vi "DMSS.main.vi"() -> ()   [LabVIEW 2014, in "DMSServer.lvlib"]
doc: "descriptionHelpStart\nThe DomainManagementServer publishes information about a CS controls domain.\n\nIt publishes four types of DIM services\n1) \"DOMAINNAME_Tasks@NODENAME\": A list of taks. Each task has a name, command line parameters and options. There is one service for each task.\n\n2) \"DOMAINNAME_CSSystems\": A list of CS systems inside the domain.\n\n3) \"DOMAINNAME_Nodes\": A list of all nodes of the domain\n\n4) \"DOMAINNAME_Info\": A service for entertaining users.\n\nFor more information please refer to\nhttp://wiki.gsi.de/cgi-bin/view/CSframework/DomainManagementSystem\ndescriptionHelpStop\n\nHistory: 16-FEB-2006, Dietrich Beck\n\nCopyright (C)\nGesellschaft für Schwerionenforschung, GSI\nPlanckstr. 1\n64291 Darmstadt\nGermany\n\nContact: D.Beck@gsi.de \n\nThis program is free software; you can redistribute it and/or modify it under the terms of the \nGNU General Public License as published by the Free Software Foundation; either version 2 of the license, or (at your option) any later version.\n\nThis program is distributed in the hope that it will be useful, but WITHOUT ANY WARRANTY; without even the implied warranty of MERCHANTABILITY or FITNESS FOR A PARTICULAR PURPOSE. See the GNU General License for more details (http://www.gnu.org).\n\nGesellschaft für Schwerionenforschung, GSI\nPlanckstr. 1, 64291 Darmstadt, Germany\nFor all questions and ideas contact D. Beck.\nLast update: 16-DEC-2005\n\n\nmenuHelpStart\nFile\n==\n- \"Load Settings\" loads a setting (*.xml) file, containing the information about a domain.\n\n- \"Save Settings\" saves the actual configuration to a setting (*.xml) file.\n\n- \"Quit (don't kill proce)\" exits this program without killing the processes marked \"kill on exit\"\n\n- \"Exit (kill procs)\" exits this program and kills the processes marked \"kill on exit\".\n\nHelp\n===\n- \"Show Description\" shows the description about this program.\n\n- \"Explain Menus\" shows this explanation\n\n- \"About LabVIEW\" shows information about LabVIEW.\n\nmenuHelpStop"
uses:
  DMSServer.lvlib
  DMSS.process_type.ctl
  DomainManagementUtils/DMSU.restart_mode.ctl
  CSlibraries/UtilityLib/UtilityLib.valueStatus.ctl
  DMSS.node_type.ctl
  CSlibraries/UtilityLib/UtilityLib.helpType.ctl
  <vilib>/Utility/xml.llb/Read From XML File(array).vi
  <vilib>/Utility/xml.llb/Write to XML File(string).vi
  CSlibraries-extern/DimLVEvent/LVDimInterface/LVDimInterface.lvlib
  DomainManagementUtils/DMSUtils.lvlib
  CSlibraries/UtilityLib/UtilityLib.lvlib
panel:
  in  "nodes":cluster{"nodeName":string, "processes":T1[]}[](array[cluster]) {"processes"."restartMode" items=["UNKNOWN", "MANUAL", "ONCE", "ALWAYS", "KILL", "SHUTDOWN"]}
  in  "updateDomain":bool
  in  "sendMessage":bool
  in  "domainMessage":string="hello world :-)\n"
  in  "Messages":i32(listbox)=-1
  in  "setDomain":bool
  in  "selectNode":u16(ring)
  in  "DomainName":string="KSTest"
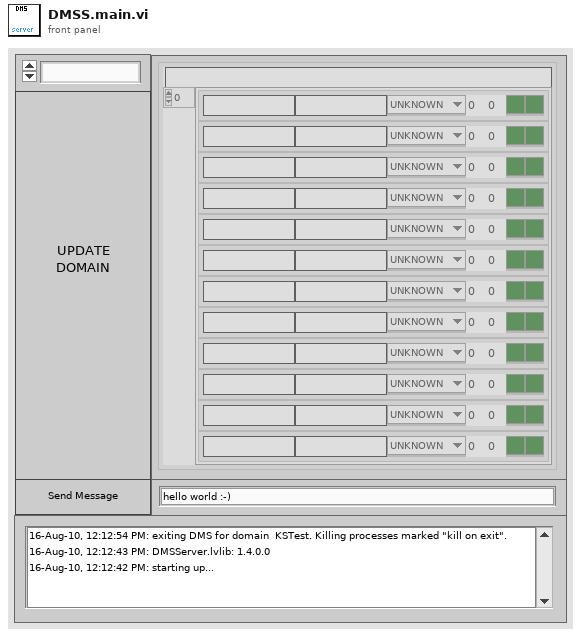
[diagram p1: front panel]
types:
  T1 = typedef "DMSServer.lvlib/DMSS.process_type.ctl" = cluster{"imageName":string, "argumentString":string, "restartMode":T2, "nOfRestart":i32, "resetRestartTimer":i32, "killOnExit":bool, "csSystem":bool}
  T2 = typedef "DMSUtils.lvlib/DMSU.restart_mode.ctl" = u16
  T3 = typedef "UtilityLib.lvlib/UtilityLib.valueStatus.ctl" = enum16{"no info available", "stand by/off", "on", "warning", "alarm/malfunction", "not implemented", "user action required", "important information", "system default", "control default", "indicator default", "button default"}
  T4 = typedef "DMSServer.lvlib/DMSS.node_type.ctl" = cluster{"nodeName":string, "processes":T1[]}
  T5 = enum16{"AddMessage", "AddErrorMessage", "GetMessages"}
  T6 = typedef "UtilityLib.lvlib/UtilityLib.helpType.ctl" = enum16{"unknown", "menu", "description", "about", "special0", "special1", "special2"}
  T7 = enum32{"invalid app kind", "Development System", "Run Time System", "Student Edition", "Embedded LabVIEW", "Evaluation", "Custom"}
  T8 = cluster{"elementBackground":u32, "elementBackground":u32}
  T9 = cluster{"elementBackground":u32, "elementBackground":u32}[]
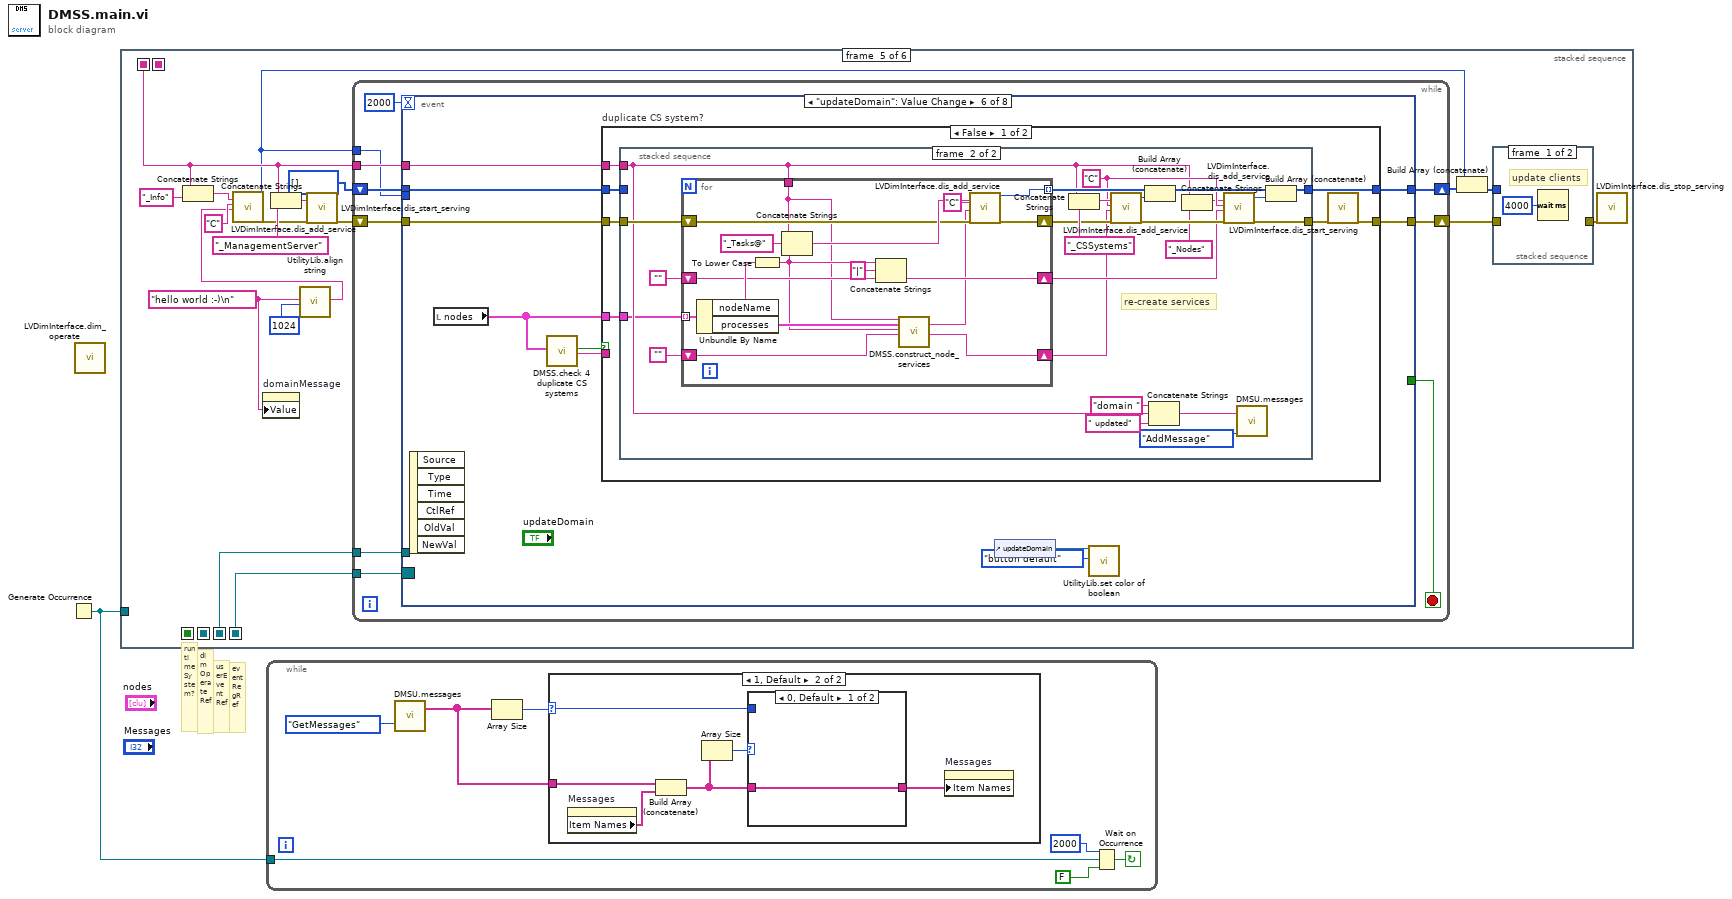
[diagram p0: block diagram]
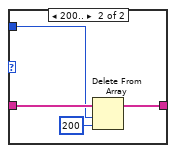
[diagram p3: hidden frame]
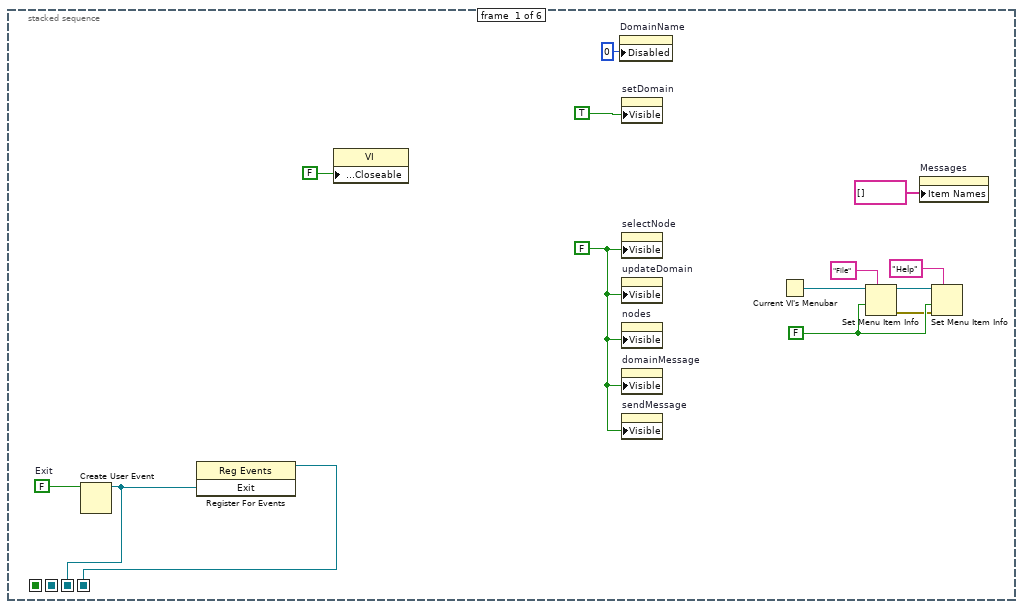
[diagram p4: hidden frame]
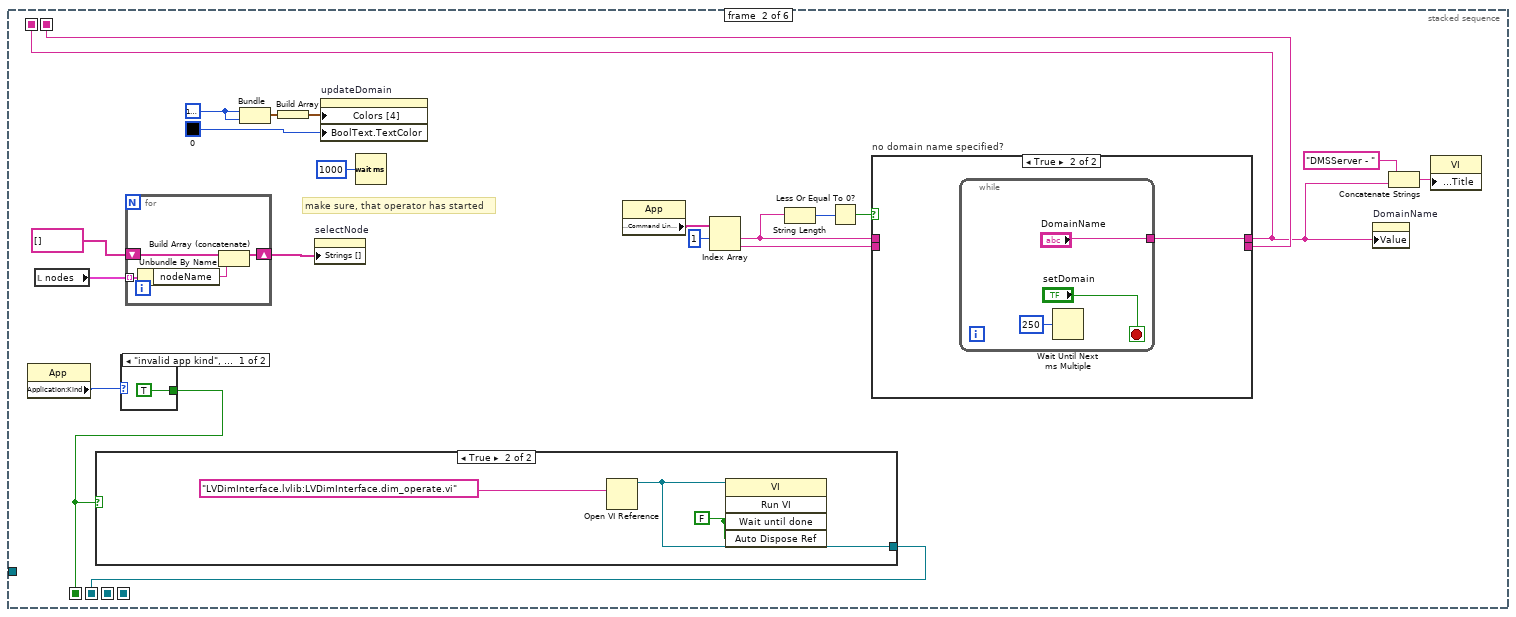
[diagram p5: hidden frame]
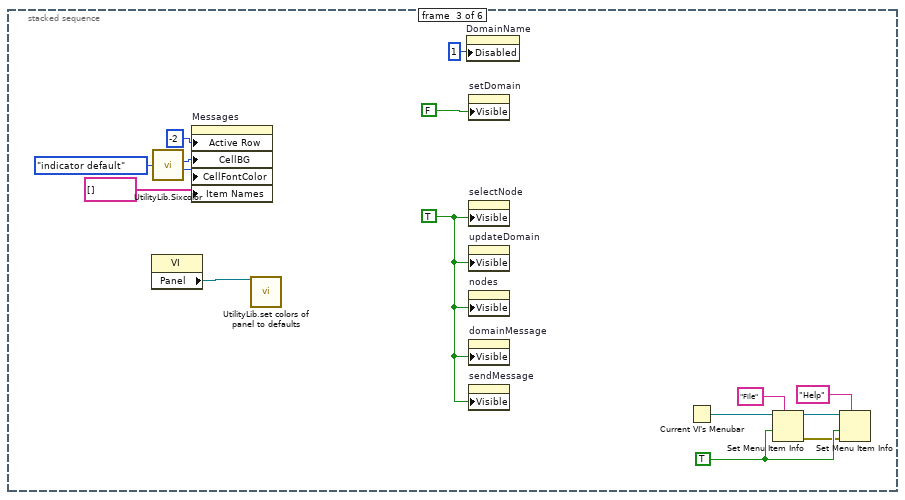
[diagram p9: hidden frame]
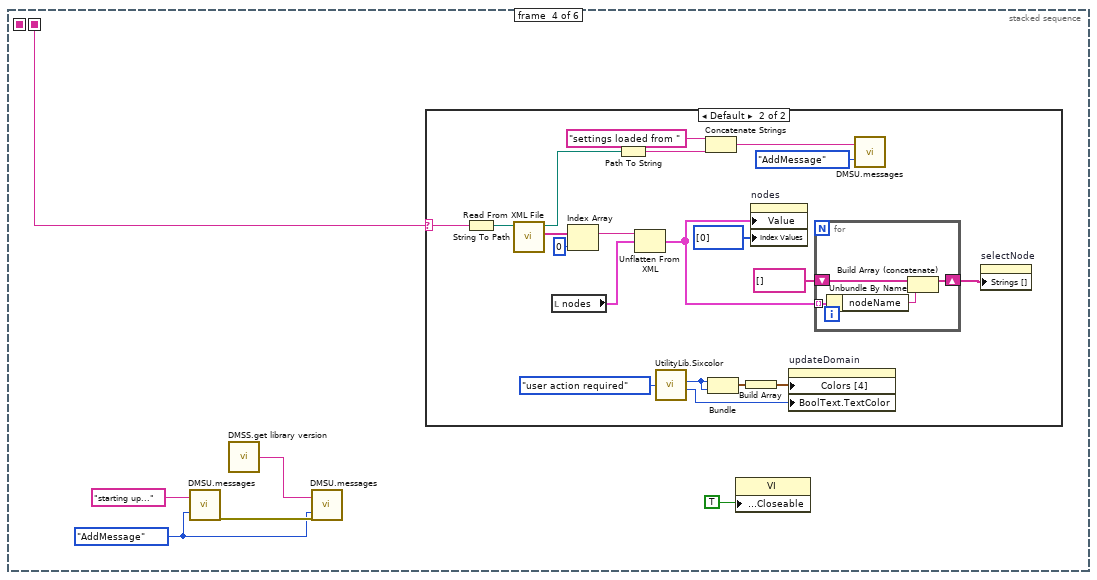
[diagram p10: hidden frame]
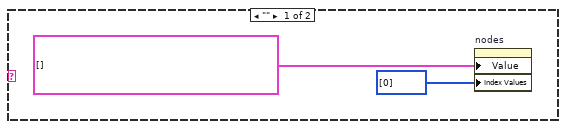
[diagram p11: hidden frame]
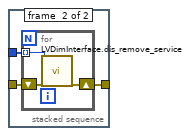
[diagram p12: hidden frame]
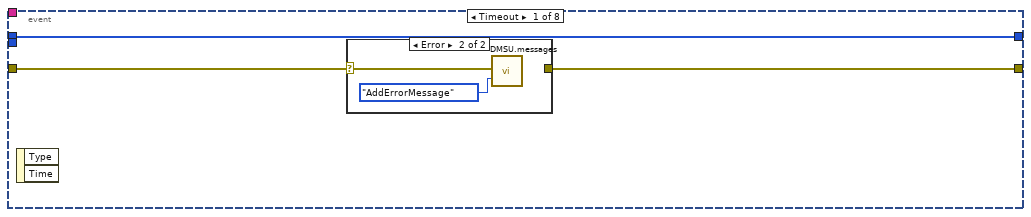
[diagram p13: hidden frame]
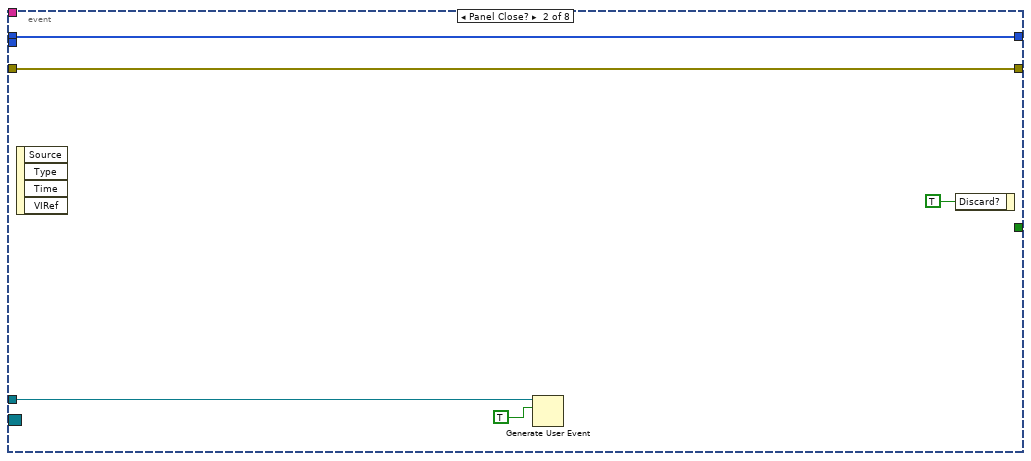
[diagram p15: hidden frame]
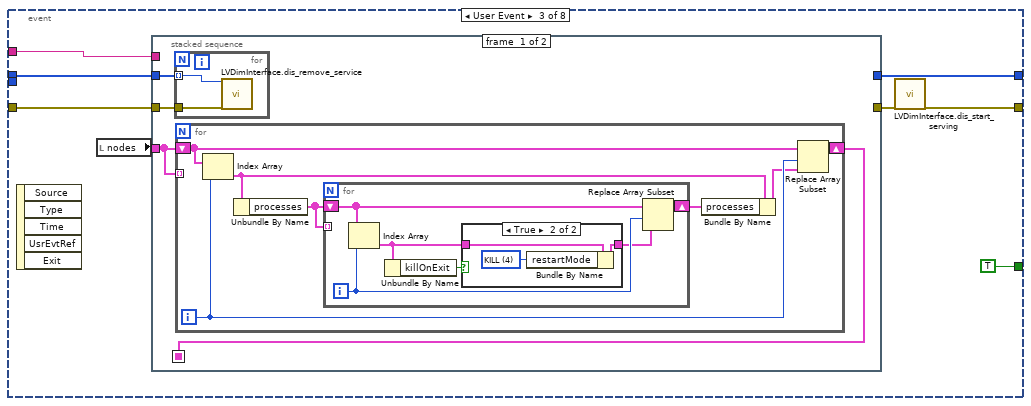
[diagram p16: hidden frame]
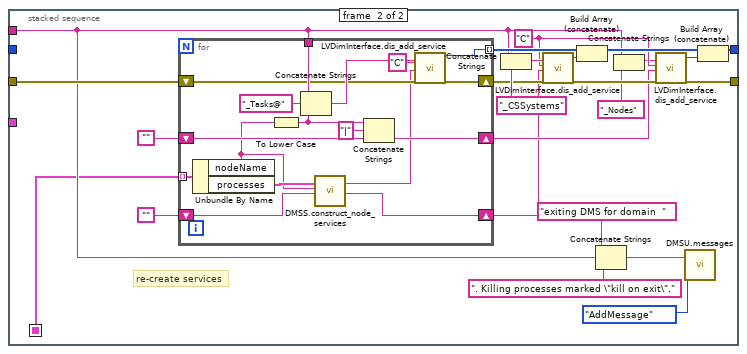
[diagram p18: hidden frame]
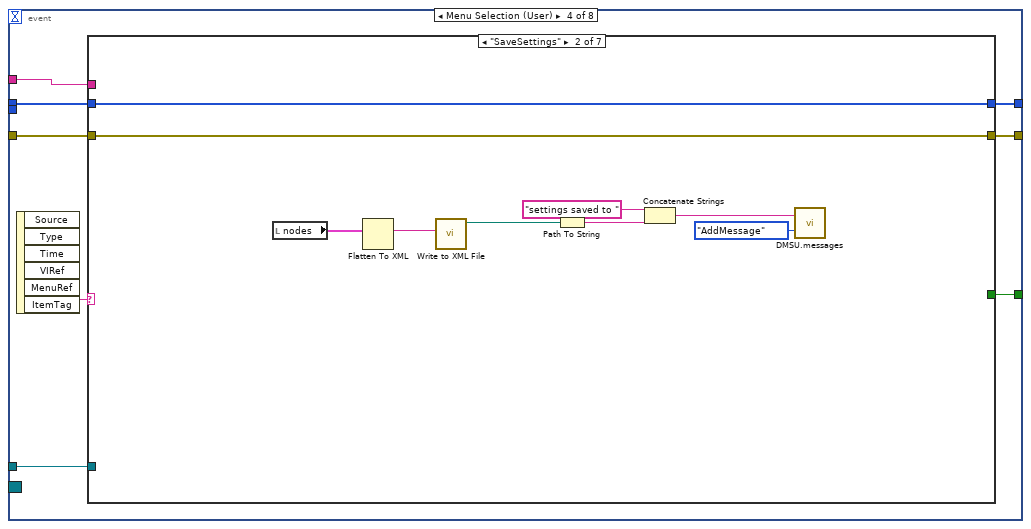
[diagram p19: hidden frame]
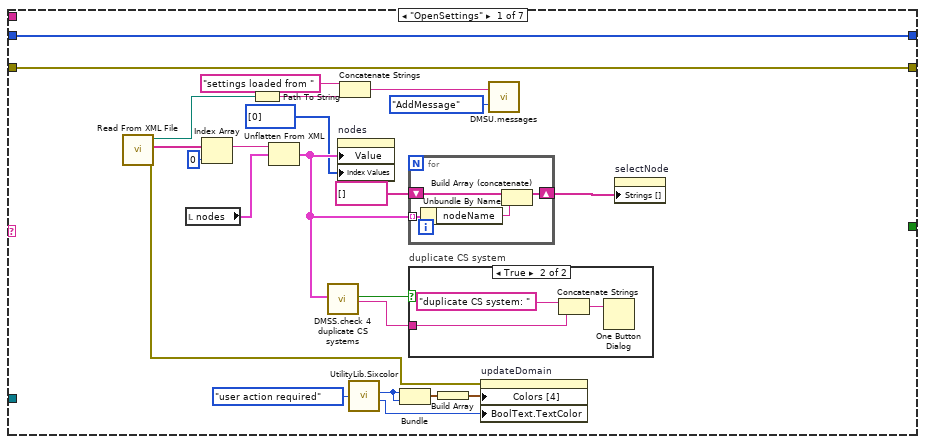
[diagram p20: hidden frame]
diagram:
  # "eventRegRef"
  # "userEventRef"
  # "dimOperateRef"
  # "runtimeSystem?"
  n1 = Generate Occurrence() -> (w1:refnum<k4>)
  n2 = call "LVDimInterface.dim_operate.vi"() -> ()  [unwired: 20 in]
  n3 = stacked-sequence {
    seq-local: [_ w20 _ _ _ _] -> [_ _ _ _ w108 _]
    seq-local: [_ w27 _ _ _ _] -> [_ _ _ _ _ w410]
    seq-local: [_ w25 _ _ _ _] -> [_ _ _ _ _ w411]
    seq-local: [_ w23 _ _ _ _] -> [_ _ _ w71 _ _]
    seq-local: [w6 _ _ _ _ _] -> [_ _ _ _ w102 _]
    seq-local: [w5 _ _ _ _ _] -> [_ _ _ _ w103 _]
    tunnel: w1 -> [_ _ _ _ _ w412]
    frame #0 {
      w7 = FALSE  # Exit
      w13 = FALSE ("enabled")
      w2 = FALSE
      n4 = Create User Event(user event datatype=w7) -> (user event=w6:refnum<user-event>)  [unwired: 1 in, 1 out]
      n5 = register-events(w6) -> (reference out=w5:refnum<event-registration>)  [unwired: 2 in, 1 out]
      n6 = property class="VI"("Front Panel.Closeable"=FALSE ("Front Panel Window:Closeable")) -> ()  [unwired: 2 in, 2 out]
      n7 = property on="DomainName" class="Str"("Disabled"=u8 0) -> ()  [unwired: 2 in, 2 out]
      n8 = property on="setDomain" class="Bool"("Visible"=TRUE) -> ()  [unwired: 2 in, 2 out]
      n9 = property on="selectNode" class="Ring (strict)"("Visible"=w2) -> ()  [unwired: 2 in, 2 out]
      n10 = property on="updateDomain" class="Bool"("Visible"=w2) -> ()  [unwired: 2 in, 2 out]
      n11 = property on="nodes" class="Arr (strict)"("Visible"=w2) -> ()  [unwired: 2 in, 2 out]
      n12 = property on="domainMessage" class="Str"("Visible"=w2) -> ()  [unwired: 2 in, 2 out]
      n13 = property on="sendMessage" class="Bool"("Visible"=w2) -> ()  [unwired: 2 in, 2 out]
      n14 = Current VI's Menubar() -> (w12:refnum<k9>)
      n15 = Set Menu Item Info(7:"File" ("item name"), 9:w13, 11:w12) -> (0:w11:errorcluster, 3:w10:refnum<k9>)  [unwired: 4 in]
      n16 = property on="Messages" class="LstBox (strict)"("Item Names"=string[] []) -> ()  [unwired: 2 in, 2 out]
      n17 = Set Menu Item Info(7:"Help" ("item name"), 8:w11, 9:w13, 11:w10) -> ()  [unwired: 3 in, 2 out]
    }
    frame #1 {
      w17 = u32 16777238 ("Color Box")
      # "make sure, that operator has started"
      n18 = property on="Property Node" class="App"() -> ("Application:Kind"=w26:T7)  [unwired: 2 in, 2 out]
      n19 = local read "nodes"() -> (w34:cluster{"nodeName":string, "processes":T1[]}[])
      n20 = case shown="\"invalid app kind\", Default" w26 {
        tunnel: [TRUE _] -> w25
        frame "invalid app kind", Default {
        }
        frame "Development System" {
        }
      }
      n21 = case shown="True" w25 {
        tunnel: [_ w39] -> w27
        frame False {
        }
        frame True {
          w40 = FALSE ("Wait until done")
          n22 = Open VI Reference(vi path="LVDimInterface.lvlib:LVDimInterface.dim_operate.vi") -> (vi reference=w39:refnum<vi>)  [unwired: 5 in, 1 out]
          n23 = invoke on="Invoke Node" class="VI" method="Run VI"(reference=w39, "Wait until done"=w40, "Auto Dispose Ref"=w40) -> ()  [unwired: 2 in, 5 out]
        }
      }
      n24 = for {
        shift-right: [w49] -> w33
        shift-left: string[] [] -> [w48]
        tunnel: w34 -> [w50] mode=indexing
        n25 = Unbundle By Name(w50) -> ("nodeName"=w47:string)
        n26 = Build Array (concatenate)(w48, w47) -> (w49:string[])
      }
      n27 = Bundle("Color Box"=w17, "Color Box"=w17) -> (w19:cluster{"Color Box":u32, "Color Box":u32})  [unwired: 1 in]
      n28 = Build Array(w19) -> (w18:cluster{"Color Box":u32, "Color Box":u32}[])
      n29 = property on="selectNode" class="Ring (strict)"("Strings []"=w33) -> ()  [unwired: 2 in, 2 out]
      n30 = property on="updateDomain" class="Bool"("Colors [4]"=w18, "BoolText.TextColor"=u32 0 ("Color Box")) -> ()  [unwired: 2 in, 2 out]
      n31 = Wait (ms)(milliseconds to wait=u32 1000) -> ()  [unwired: 1 out]
      n32 = property on="Property Node" class="App"() -> ("Application:Command Line Arguments"=w32:string[])  [unwired: 2 in, 2 out]
      n33 = Index Array(array=w32, index #1=1 ("index")) -> (element #1=w28:string, element #2=w24:string)  [unwired: 1 in]
      n34 = String Length(string=w28) -> (length=w30:i32)
      n35 = Less Or Equal To 0?(x=w30) -> (x <= 0?=w29:bool)
      n36 = case "no domain name specified?" shown="True" w29 {
        tunnel: [w42 w43] -> w20
        tunnel: w28 -> [w42 _]
        tunnel: [w41 _] -> w23
        tunnel: w24 -> [w41 _]
        frame False {
        }
        frame True {
          n37 = while {
            tunnel: ["DomainName"] -> w43
            stop <- "setDomain" stop-if-true
            n38 = Wait Until Next ms Multiple(millisecond multiple=u32 250) -> ()  [unwired: 1 out]
          }
        }
      }
      n39 = property on="DomainName" class="Str"("Value"=w20) -> ()  [unwired: 2 in, 2 out]
      n40 = Concatenate Strings("DMSServer - " ("string"), w20) -> (w22:string)
      n41 = property on="Property Node" class="VI"("Front Panel.Title"=w22) -> ()  [unwired: 2 in, 2 out]
    }
    frame #2 {
      w64 = TRUE ("enabled")
      w51 = TRUE
      n42 = property on="Property Node" class="VI"() -> ("Panel"=w53:refnum<vi>)  [unwired: 2 in, 2 out]
      n43 = call "UtilityLib.Sixcolor.vi"("State"=UtilityLib.valueStatus."indicator default") -> ("elementBackground"=w57:u32, "elementText"=w56:u32)  [unwired: 2 in, 2 out]
      n44 = property on="Messages" class="LstBox (strict)"("Active Row"=-2 ("Active Row:Active Row Number"), "CellBG"=w57, "CellFontColor"=w56, "Item Names"=string[] []) -> ()  [unwired: 2 in, 2 out]
      n45 = call "UtilityLib.set colors of panel to defaults.vi"("Front Panel"=w53) -> ()  [unwired: 18 in, 1 out]
      n46 = property on="DomainName" class="Str"("Disabled"=u8 1) -> ()  [unwired: 2 in, 2 out]
      n47 = property on="setDomain" class="Bool"("Visible"=FALSE) -> ()  [unwired: 2 in, 2 out]
      n48 = property on="selectNode" class="Ring (strict)"("Visible"=w51) -> ()  [unwired: 2 in, 2 out]
      n49 = property on="updateDomain" class="Bool"("Visible"=w51) -> ()  [unwired: 2 in, 2 out]
      n50 = property on="nodes" class="Arr (strict)"("Visible"=w51) -> ()  [unwired: 2 in, 2 out]
      n51 = property on="domainMessage" class="Str"("Visible"=w51) -> ()  [unwired: 2 in, 2 out]
      n52 = property on="sendMessage" class="Bool"("Visible"=w51) -> ()  [unwired: 2 in, 2 out]
      n53 = Current VI's Menubar() -> (w63:refnum<k9>)
      n54 = Set Menu Item Info(7:"File" ("item name"), 9:w64, 11:w63) -> (0:w62:errorcluster, 3:w61:refnum<k9>)  [unwired: 4 in]
      n55 = Set Menu Item Info(7:"Help" ("item name"), 8:w62, 9:w64, 11:w61) -> ()  [unwired: 3 in, 2 out]
    }
    frame #3 {
      w66 = T5."AddMessage" ("Action")
      n56 = call "DMSU.messages.vi"("message"="starting up...", "Action"=w66) -> ("error out"=w68:errorcluster)  [unwired: 16 in, 1 out]
      n57 = call "DMSS.get library version.vi"() -> ("nameAndVersion"=w67:string)  [unwired: 1 in]
      n58 = call "DMSU.messages.vi"("message"=w67, "Action"=w66, "error in (no error)"=w68) -> ()  [unwired: 15 in, 2 out]
      n59 = case shown="Default" w71 {
        selector: w71 -> [_ w81]
        frame "" {
          n60 = property on="nodes" class="Arr (strict)"("Value"=T4[] [] ("nodes"), "Index Values"=u32[] [0]) -> ()  [unwired: 2 in, 2 out]
        }
        frame Default {
          n61 = String To Path(string=w81) -> (path=w82:path)
          n62 = call-poly <vilib>:"Read From XML File.vi"("XML File Path"=w82) -> ("XML Elements"=w93:string[], "XML File Path(duplicate)"=w83:path)  [unwired: 8 in, 1 out]
          n63 = local read "nodes"() -> (w88:cluster{"nodeName":string, "processes":T1[]}[])
          n64 = Index Array(array=w93, index=0) -> (element=w91:string)
          n65 = Path To String(path=w83) -> (string=w85:string)
          n66 = Unflatten From XML(xml string=w91, type=w88) -> (value=w74:cluster{"nodeName":string, "processes":T1[]}[])  [unwired: 1 in, 1 out]
          n67 = call "UtilityLib.Sixcolor.vi"("State"=UtilityLib.valueStatus."user action required") -> ("elementBackground"=w77:u32, "elementText"=w76:u32)  [unwired: 2 in, 2 out]
          n68 = Concatenate Strings("settings loaded from " ("message"), w85) -> (w84:string)
          n69 = Bundle("elementBackground"=w77, "elementBackground"=w77) -> (w79:T8)  [unwired: 1 in]
          n70 = Build Array(w79) -> (w78:T9)
          n71 = property on="nodes" class="Arr (strict)"("Value"=w74, "Index Values"=u32[] [0]) -> ()  [unwired: 2 in, 2 out]
          n72 = property on="updateDomain" class="Bool"("Colors [4]"=w78, "BoolText.TextColor"=w76) -> ()  [unwired: 2 in, 2 out]
          n73 = for {
            shift-right: [w96] -> w89
            shift-left: string[] [] -> [w95]
            tunnel: w74 -> [w97] mode=indexing
            n74 = Unbundle By Name(w97) -> ("nodeName"=w94:string)
            n75 = Build Array (concatenate)(w95, w94) -> (w96:string[])
          }
          n76 = call "DMSU.messages.vi"("message"=w84, "Action"=T5."AddMessage") -> ()  [unwired: 16 in, 2 out]
          n77 = property on="selectNode" class="Ring (strict)"("Strings []"=w89) -> ()  [unwired: 2 in, 2 out]
        }
      }
      n78 = property class="VI"("Front Panel.Closeable"=TRUE ("Front Panel Window:Closeable")) -> ()  [unwired: 2 in, 2 out]
    }
    frame #4 {
      w98 = "hello world :-)\n" ("data")
      n79 = Concatenate Strings(w108, "_Info" ("string")) -> (w110:string)
      n80 = property on="domainMessage" class="Str"("Value"=w98) -> ()  [unwired: 2 in, 2 out]
      n81 = Concatenate Strings(w108, "_ManagementServer" ("string")) -> (w116:string)
      n82 = call "UtilityLib.align string.vi"("stringIn"=w98, "stringLength (80)"=u16 1024) -> ("stringOut"=w100:string)  [unwired: 16 in, 1 out]
      n83 = call "LVDimInterface.dis_add_service.vi"("serviceName"=w110, "typeDescriptor"="C", "data"=w100) -> ("my_serviceID"=w101:i32, "error out"=w107:errorcluster)  [unwired: 15 in]
      n84 = call "LVDimInterface.dis_start_serving.vi"("serverName"=w116, "error in (no error)"=w107) -> ("error out"=w114:errorcluster)  [unwired: 16 in, 1 out]
      n85 = while {
        tunnel: w108 -> [w130]
        shift-right: [w129] -> w105
        shift-left: i32[] [] -> [w128]
        shift-right: [w131] -> w113
        shift-left: w114 -> [w132]
        tunnel: w103 -> [w126]
        tunnel: w102 -> [w125]
        tunnel: w101 -> [w124]
        stop <- w133 stop-if-true
        n86 = event shown="[5] \"updateDomain\": Value Change" {
          selector: w126 -> [_ _ _ _ _ _ _ _]
          dyn-events: _ -> [_ _ _ _ _ _ _ _]
          timeout: 2000 -> [_ _ _ _ _ _ _ _]
          tunnel: [_ _ TRUE w219 _ _ _ _] -> w133
          tunnel: w132 -> [w135 w142 w147 w220 w288 w305 w367 w382]
          tunnel: [w134 w142 w145 w221 w288 w304 w367 w375] -> w131
          tunnel: w130 -> [_ _ w149 w218 _ w308 _ _]
          tunnel: [w136 w143 w146 w222 w291 w307 w368 w373] -> w129
          tunnel: w128 -> [w136 w143 w148 w223 w291 w306 w368 w374]
          tunnel: w125 -> [_ w140 _ w217 _ _ _ _]
          tunnel: w124 -> [_ _ _ _ _ _ _ w383]
          event Timeout {
            n87 = event-data() -> ()  [unwired: 1 in, 2 out]
            n88 = case shown="Error" w135 {
              selector: w135 -> [w137 w139]
              tunnel: [w137 _] -> w134
              frame No Error {
              }
              frame Error {
                n89 = call "DMSU.messages.vi"("errorMessage"=w139, "Action"=T5."AddErrorMessage") -> ()  [unwired: 16 in, 2 out]
              }
            }
          }
          event Panel Close? {
            n90 = event-data() -> ()  [unwired: 1 in, 4 out]
            n91 = Generate User Event(user event=w140, event data cluster=TRUE ("event data")) -> ()  [unwired: 2 in, 2 out]
            n92 = event-data ("Event Filter Node")("Discard?"=TRUE) -> ()  [unwired: 1 in, 1 out]
          }
          event User Event {
            n93 = event-data() -> ()  [unwired: 1 in, 5 out]
            n94 = local read "nodes"() -> (w150:cluster{"nodeName":string, "processes":T1[]}[])
            n95 = stacked-sequence {
              seq-local: [w153 _] -> [_ w176]
              tunnel: w149 -> [_ w177]
              tunnel: [_ w187] -> w146
              tunnel: w148 -> [w156 _]
              tunnel: [_ w190] -> w151
              tunnel: w147 -> [w155 w198]
              tunnel: w150 -> [w154 _]
              frame #0 {
                n96 = for {
                  tunnel: w156 -> [w175] mode=indexing
                  tunnel: w155 -> [w174]
                  n97 = call "LVDimInterface.dis_remove_service.vi"("my_serviceID"=w175, "error in (no error)"=w174) -> ()  [unwired: 17 in, 1 out]
                }
                n98 = for {
                  tunnel: w154 -> [_] mode=indexing
                  shift-right: [w161] -> w153
                  shift-left: w154 -> [w162]
                  i -> [w160]
                  n99 = Index Array(array=w162, index=w160) -> (element=w159:cluster{"nodeName":string, "processes":T1[]})
                  n100 = Unbundle By Name(w159) -> ("processes"=w163:T1[])
                  n101 = for {
                    tunnel: w163 -> [_] mode=indexing
                    shift-right: [w164] -> w158
                    shift-left: w163 -> [w168]
                    i -> [w167]
                    n102 = Index Array(array=w168, index=w167) -> (element=w166:T1)
                    n103 = Unbundle By Name(w166) -> ("killOnExit"=w169:bool)
                    n104 = case shown="True" w169 {
                      tunnel: [w170 w172] -> w165
                      tunnel: w166 -> [w170 w173]
                      frame False {
                      }
                      frame True {
                        w171 = T2 4 items=["UNKNOWN", "MANUAL", "ONCE", "ALWAYS", "KILL"] ("restartMode")
                        n105 = Bundle By Name(cluster=w173, "restartMode"=w171) -> (w172:T1)
                      }
                    }
                    n106 = Replace Array Subset(array=w168, new element=w165, index=w167) -> (w164:T1[])
                  }
                  n107 = Bundle By Name(cluster=w159, "processes"=w158) -> (w157:cluster{"nodeName":string, "processes":T1[]})
                  n108 = Replace Array Subset(array=w162, new element=w157, index=w160) -> (w161:cluster{"nodeName":string, "processes":T1[]}[])
                }
              }
              frame #1 {
                w184 = "C" ("typeDescriptor")
                # "re-create services"
                n109 = for {
                  tunnel: w176 -> [w216] mode=indexing
                  tunnel: w177 -> [w215]
                  tunnel: [w211] -> w194 mode=indexing
                  shift-right: [w201] -> w182
                  shift-left: "" ("Empty String Constant") -> [w202]
                  shift-right: [w210] -> w195
                  shift-left: w198 -> [w209]
                  shift-right: [w205] -> w185
                  shift-left: "" ("Empty String Constant") -> [w206]
                  n110 = Unbundle By Name(w216) -> ("nodeName"=w200:string, "processes"=w204:T1[])
                  n111 = To Lower Case(string=w200) -> (all lower case string=w207:string)
                  n112 = Concatenate Strings(w215, "_Tasks@" ("string"), w207) -> (w213:string)
                  n113 = call "DMSS.construct_node_services.vi"("processes"=w204, "nodeName"=w200, "CSSystems"=w202) -> ("taskList"=w203:string, "CSSystems (out)"=w201:string)  [unwired: 15 in]
                  n114 = Concatenate Strings(w207, "|" ("string"), w206) -> (w205:string)
                  n115 = call "LVDimInterface.dis_add_service.vi"("serviceName"=w213, "typeDescriptor"="C", "data"=w203, "error in (no error)"=w209) -> ("my_serviceID"=w211:i32, "error out"=w210:errorcluster)  [unwired: 14 in]
                }
                n116 = Concatenate Strings(w177, "_CSSystems" ("string")) -> (w196:string)
                n117 = call "LVDimInterface.dis_add_service.vi"("serviceName"=w196, "typeDescriptor"=w184, "data"=w182, "error in (no error)"=w195) -> ("my_serviceID"=w193:i32, "error out"=w191:errorcluster)  [unwired: 14 in]
                n118 = Build Array (concatenate)(w194, w193) -> (w188:i32[])
                n119 = Concatenate Strings("exiting DMS for domain  " ("string"), w177, ". Killing processes marked \"kill on exit\"." ("string")) -> (w178:string)
                n120 = Concatenate Strings(w177, "_Nodes" ("string")) -> (w183:string)
                n121 = call "LVDimInterface.dis_add_service.vi"("serviceName"=w183, "typeDescriptor"=w184, "data"=w185, "error in (no error)"=w191) -> ("my_serviceID"=w189:i32, "error out"=w190:errorcluster)  [unwired: 14 in]
                n122 = call "DMSU.messages.vi"("message"=w178, "Action"=T5."AddMessage") -> ()  [unwired: 16 in, 2 out]
                n123 = Build Array (concatenate)(w188, w189) -> (w187:i32[])
              }
            }
            n124 = call "LVDimInterface.dis_start_serving.vi"("error in (no error)"=w151) -> ("error out"=w145:errorcluster)  [unwired: 17 in, 1 out]
          }
          event Menu Selection (User) {
            n125 = event-data() -> ("ItemTag"=w224:string)  [unwired: 1 in, 5 out]
            n126 = case shown="\"SaveSettings\"" w224 {
              tunnel: w223 -> [w235 w256 w265 w270 w272 w275 w278]
              tunnel: [w235 w256 w265 w270 w272 w275 w278] -> w222
              tunnel: w220 -> [w234 w255 w264 w269 w271 w274 w277]
              tunnel: [w234 w255 w264 w269 w271 w274 w277] -> w221
              tunnel: [_ _ TRUE _ _ _ _] -> w219
              tunnel: w218 -> [_ _ _ _ _ _ _]
              tunnel: w217 -> [_ _ _ w267 _ _ _]
              frame "OpenSettings" {
                n127 = call-poly <vilib>:"Read From XML File.vi"() -> ("error out"=w229:errorcluster, "XML Elements"=w247:string[], "XML File Path(duplicate)"=w238:path)  [unwired: 9 in]
                n128 = local read "nodes"() -> (w243:cluster{"nodeName":string, "processes":T1[]}[])
                n129 = Index Array(array=w247, index=0) -> (element=w245:string)
                n130 = Path To String(path=w238) -> (string=w240:string)
                n131 = Unflatten From XML(xml string=w245, type=w243) -> (value=w226:cluster{"nodeName":string, "processes":T1[]}[])  [unwired: 1 in, 1 out]
                n132 = call "DMSS.check 4 duplicate CS systems.vi"("Nodes"=w226) -> ("duplicateSystem"=w237:bool, "systemName"=w236:string)  [unwired: 17 in]
                n133 = property on="nodes" class="Arr (strict)"("Value"=w226, "Index Values"=u32[] [0]) -> ()  [unwired: 2 in, 2 out]
                n134 = Concatenate Strings("settings loaded from " ("message"), w240) -> (w239:string)
                n135 = call "UtilityLib.Sixcolor.vi"("State"=UtilityLib.valueStatus."user action required") -> ("elementBackground"=w230:u32, "elementText"=w228:u32)  [unwired: 2 in, 2 out]
                n136 = Bundle("elementBackground"=w230, "elementBackground"=w230) -> (w232:T8)  [unwired: 1 in]
                n137 = for {
                  shift-right: [w253] -> w244
                  shift-left: string[] [] -> [w252]
                  tunnel: w226 -> [w254] mode=indexing
                  n138 = Unbundle By Name(w254) -> ("nodeName"=w251:string)
                  n139 = Build Array (concatenate)(w252, w251) -> (w253:string[])
                }
                n140 = case "duplicate CS system" shown="True" w237 {
                  tunnel: w236 -> [_ w250]
                  frame False {
                  }
                  frame True {
                    n141 = Concatenate Strings("duplicate CS system: " ("string"), w250) -> (w248:string)
                    n142 = One Button Dialog(message=w248) -> ()  [unwired: 1 in, 1 out]
                  }
                }
                n143 = Build Array(w232) -> (w231:T9)
                n144 = property on="updateDomain" class="Bool"(error in=w229, "Colors [4]"=w231, "BoolText.TextColor"=w228) -> ()  [unwired: 1 in, 2 out]
                n145 = call "DMSU.messages.vi"("message"=w239, "Action"=T5."AddMessage") -> ()  [unwired: 16 in, 2 out]
                n146 = property on="selectNode" class="Ring (strict)"("Strings []"=w244) -> ()  [unwired: 2 in, 2 out]
              }
              frame "SaveSettings" {
                n147 = local read "nodes"() -> (w263:cluster{"nodeName":string, "processes":T1[]}[])
                n148 = Flatten To XML(anything=w263) -> (xml string=w262:string)
                n149 = call-poly <vilib>:"Write to XML File.vi"("XML Input"=w262) -> ("XML File Path(duplicate)"=w259:path)  [unwired: 8 in, 2 out]
                n150 = Path To String(path=w259) -> (string=w258:string)
                n151 = Concatenate Strings("settings saved to " ("message"), w258) -> (w257:string)
                n152 = call "DMSU.messages.vi"("message"=w257, "Action"=T5."AddMessage") -> ()  [unwired: 16 in, 2 out]
              }
              frame "Quit" {
              }
              frame "Exit" {
                n153 = Generate User Event(user event=w267, event data cluster=TRUE ("event data")) -> ()  [unwired: 2 in, 2 out]
              }
              frame "ExplainMenus" {
                n154 = call "UtilityLib.show help.vi"("helpType"=UtilityLib.helpType."menu") -> ()
              }
              frame "ShowDescription" {
                n155 = call "UtilityLib.show help.vi"("helpType"=UtilityLib.helpType."description") -> ()
              }
              frame Default {
              }
            }
          }
          event "nodes": Value Change {
            # "DN: This should be enough to\nsort the node array\nAll links should be still working"
            n156 = event-data() -> ()  [unwired: 1 in, 6 out]
            n157 = local read "nodes"() -> (w280:cluster{"nodeName":string, "processes":T1[]}[])
            n158 = Sort 1D Array(array=w280) -> (sorted array=w279:cluster{"nodeName":string, "processes":T1[]}[])
            n159 = call "UtilityLib.Sixcolor.vi"("State"=UtilityLib.valueStatus."user action required") -> ("elementBackground"=w282:u32, "elementText"=w281:u32)  [unwired: 2 in, 2 out]
            n160 = local write "nodes"(w279) -> ()
            n161 = Bundle("elementBackground"=w282, "elementBackground"=w282) -> (w284:T8)  [unwired: 1 in]
            n162 = Build Array(w284) -> (w283:T9)
            n163 = property on="updateDomain" class="Bool"("Colors [4]"=w283, "BoolText.TextColor"=w281) -> ()  [unwired: 2 in, 2 out]
            n164 = call "DMSS.check 4 duplicate CS systems.vi"("Nodes"=w279) -> ("duplicateSystem"=w287:bool, "systemName"=w286:string)  [unwired: 17 in]
            n165 = for {
              shift-right: [w297] -> w289
              shift-left: string[] [] -> [w296]
              tunnel: w279 -> [w298] mode=indexing
              n166 = Unbundle By Name(w298) -> ("nodeName"=w295:string)
              n167 = Build Array (concatenate)(w296, w295) -> (w297:string[])
            }
            n168 = case "duplicate CS system" shown="True" w287 {
              tunnel: w286 -> [_ w294]
              frame False {
              }
              frame True {
                n169 = Concatenate Strings("duplicate CS system: " ("string"), w294) -> (w292:string)
                n170 = One Button Dialog(message=w292) -> ()  [unwired: 1 in, 1 out]
              }
            }
            n171 = property on="selectNode" class="Ring (strict)"("Strings []"=w289) -> ()  [unwired: 2 in, 2 out]
          }
          event "updateDomain": Value Change {
            n172 = event-data() -> ()  [unwired: 1 in, 6 out]
            n173 = local read "nodes"() -> (w303:cluster{"nodeName":string, "processes":T1[]}[])
            n174 = call "DMSS.check 4 duplicate CS systems.vi"("Nodes"=w303) -> ("duplicateSystem"=w302:bool, "systemName"=w301:string)  [unwired: 17 in]
            n175 = case "duplicate CS system?" shown="False" w302 {
              tunnel: w308 -> [w315 _]
              tunnel: [w314 w362] -> w307
              tunnel: w306 -> [w313 w362]
              tunnel: w305 -> [w312 w361]
              tunnel: [w311 w361] -> w304
              tunnel: w303 -> [w309 _]
              tunnel: w301 -> [_ w363]
              frame False {
                n176 = stacked-sequence {
                  tunnel: w315 -> [_ w321]
                  tunnel: [_ w331] -> w314
                  tunnel: w313 -> [w317 _]
                  tunnel: [_ w334] -> w310
                  tunnel: w312 -> [w316 w342]
                  tunnel: w309 -> [_ w320]
                  frame #0 {
                    # "remove services"
                    n177 = for {
                      tunnel: w317 -> [w319] mode=indexing
                      tunnel: w316 -> [w318]
                      n178 = call "LVDimInterface.dis_remove_service.vi"("my_serviceID"=w319, "error in (no error)"=w318) -> ()  [unwired: 17 in, 1 out]
                    }
                  }
                  frame #1 {
                    w328 = "C" ("typeDescriptor")
                    # "re-create services"
                    n179 = for {
                      tunnel: w320 -> [w360] mode=indexing
                      tunnel: w321 -> [w344]
                      tunnel: [w355] -> w338 mode=indexing
                      shift-right: [w346] -> w326
                      shift-left: "" ("Empty String Constant") -> [w347]
                      shift-right: [w354] -> w339
                      shift-left: w342 -> [w353]
                      shift-right: [w350] -> w329
                      shift-left: "" ("Empty String Constant") -> [w351]
                      n180 = Unbundle By Name(w360) -> ("nodeName"=w359:string, "processes"=w349:T1[])
                      n181 = To Lower Case(string=w359) -> (all lower case string=w345:string)
                      n182 = Concatenate Strings(w344, "_Tasks@" ("string"), w345) -> (w357:string)
                      n183 = Concatenate Strings(w345, "|" ("string"), w351) -> (w350:string)
                      n184 = call "DMSS.construct_node_services.vi"("domainName"=w344, "processes"=w349, "nodeName"=w345, "CSSystems"=w347) -> ("taskList"=w348:string, "CSSystems (out)"=w346:string)  [unwired: 14 in]
                      n185 = call "LVDimInterface.dis_add_service.vi"("serviceName"=w357, "typeDescriptor"="C", "data"=w348, "error in (no error)"=w353) -> ("my_serviceID"=w355:i32, "error out"=w354:errorcluster)  [unwired: 14 in]
                    }
                    n186 = Concatenate Strings(w321, "_CSSystems" ("string")) -> (w340:string)
                    n187 = call "LVDimInterface.dis_add_service.vi"("serviceName"=w340, "typeDescriptor"=w328, "data"=w326, "error in (no error)"=w339) -> ("my_serviceID"=w337:i32, "error out"=w335:errorcluster)  [unwired: 14 in]
                    n188 = Build Array (concatenate)(w338, w337) -> (w332:i32[])
                    n189 = Concatenate Strings("domain " ("string"), w321, " updated" ("string")) -> (w322:string)
                    n190 = Concatenate Strings(w321, "_Nodes" ("string")) -> (w327:string)
                    n191 = call "LVDimInterface.dis_add_service.vi"("serviceName"=w327, "typeDescriptor"=w328, "data"=w329, "error in (no error)"=w335) -> ("my_serviceID"=w333:i32, "error out"=w334:errorcluster)  [unwired: 14 in]
                    n192 = call "DMSU.messages.vi"("message"=w322, "Action"=T5."AddMessage") -> ()  [unwired: 16 in, 2 out]
                    n193 = Build Array (concatenate)(w332, w333) -> (w331:i32[])
                  }
                }
                n194 = call "LVDimInterface.dis_start_serving.vi"("error in (no error)"=w310) -> ("error out"=w311:errorcluster)  [unwired: 17 in, 1 out]
              }
              frame True {
                n195 = Concatenate Strings("refusing update - duplicate CS system: " ("string"), w363) -> (w364:string)
                n196 = One Button Dialog(message=w364) -> ()  [unwired: 1 in, 1 out]
              }
            }
            n197 = control-ref of="updateDomain"() -> (w300:refnum<vi>)
            n198 = call "UtilityLib.set color of boolean.vi"("button"=w300, "valueStatus"=UtilityLib.valueStatus."button default") -> ()  [unwired: 17 in, 1 out]
          }
          event "selectNode": Value Change {
            n199 = event-data() -> ()  [unwired: 1 in, 6 out]
            n200 = Build Array("selectNode") -> (w366:u16[])
            n201 = property on="nodes" class="Arr (strict)"("Index Values"=w366) -> ()  [unwired: 2 in, 2 out]
          }
          event "sendMessage": Value Change {
            n202 = event-data() -> ()  [unwired: 1 in, 6 out]
            n203 = Concatenate Strings("domainMessage", "\n" ("string")) -> (w372:string)
            n204 = call "UtilityLib.align string.vi"("stringIn"=w372, "stringLength (80)"=u16 1024) -> ("stringOut"=w371:string)  [unwired: 16 in, 1 out]
            n205 = call "LVDimInterface.dis_update_service.vi"("my_serviceID"=w383, "data"=w371, "error in (no error)"=w382) -> ("my_serviceID out"=w377:i32, "error out"=w376:errorcluster)  [unwired: 14 in, 1 out]
            n206 = Match Pattern(string=w371, regular expression="SHUTDOWN") -> (offset past match=w378:i32)  [unwired: 1 in, 3 out]
            n207 = case "shutdown message?" shown="0, Default" w378 {
              tunnel: w377 -> [w388 _]
              tunnel: w376 -> [w387 w409]
              tunnel: w371 -> [w389 _]
              tunnel: [w386 w409] -> w375
              tunnel: w374 -> [w385 w408]
              tunnel: [w384 w408] -> w373
              frame 0, Default {
                n208 = Wait (ms)(milliseconds to wait=u32 2000) -> (millisecond timer value=w390:u32)
                n209 = Two Button Dialog(message="Remove shutdown message to avoid repeated shutdowns?", 1:"No" ("F button name (\"Cancel\")"), 2:"Yes" ("T button name (\"OK\")")) -> (T button?=w394:bool)
                n210 = case "remove shutdown message?" shown="True" w394 {
                  tunnel: w390 -> [_ _]
                  tunnel: w389 -> [_ w405]
                  tunnel: w388 -> [_ w407]
                  tunnel: w387 -> [w397 w406]
                  tunnel: [w397 w403] -> w386
                  tunnel: [w396 w402] -> w384
                  tunnel: w385 -> [w396 w402]
                  frame False {
                  }
                  frame True {
                    n211 = Concatenate Strings("was: " ("string"), w405) -> (w401:string)
                    n212 = call "UtilityLib.align string.vi"("stringIn"=w401, "stringLength (80)"=u16 1024) -> ("stringOut"=w399:string)  [unwired: 16 in, 1 out]
                    n213 = call "UtilityLib.remove white spaces.vi"("string with blanks"=w399) -> ("string without white spaces"=w398:string)  [unwired: 14 in, 4 out]
                    n214 = call "LVDimInterface.dis_update_service.vi"("my_serviceID"=w407, "data"=w399, "error in (no error)"=w406) -> ("error out"=w403:errorcluster)  [unwired: 14 in, 2 out]
                    n215 = property on="domainMessage" class="Str"("Value"=w398) -> ()  [unwired: 2 in, 2 out]
                  }
                }
              }
              frame -1 {
              }
            }
          }
        }
      }
      n216 = Build Array (concatenate)(w101, w105) -> (w104:i32[])
      n217 = stacked-sequence {
        tunnel: w104 -> [_ w120]
        tunnel: w113 -> [_ w119]
        tunnel: [_ w118] -> w112
        frame #0 {
          # "update clients"
          n218 = Wait (ms)(milliseconds to wait=u32 4000) -> ()  [unwired: 1 out]
        }
        frame #1 {
          n219 = for {
            tunnel: w120 -> [w123] mode=indexing
            shift-right: [w121] -> w118
            shift-left: w119 -> [w122]
            n220 = call "LVDimInterface.dis_remove_service.vi"("my_serviceID"=w123, "error in (no error)"=w122) -> ("error out"=w121:errorcluster)  [unwired: 17 in]
          }
        }
      }
      n221 = call "LVDimInterface.dis_stop_serving.vi"("error in (no error)"=w112) -> ()  [unwired: 18 in, 1 out]
    }
    frame #5 {
      n222 = Set Occurrence(w412) -> ()
      n223 = case shown="True" w411 {
        tunnel: w410 -> [_ w417]
        frame False {
        }
        frame True {
          n224 = invoke on="Invoke Node" class="VI" method="Ctrl Val.Set"(reference=w417, "Control Name"="stop", "Value"=TRUE) -> (error out=w419:errorcluster)  [unwired: 2 in, 4 out]
          n225 = flat-sequence {
            tunnel: w417 -> [w422]
            tunnel: w419 -> [w423]
            tunnel: [w423] -> w416
            tunnel: [w422] -> w415
            tunnel: w416 -> [w425]
            tunnel: w415 -> [w424]
            frame #0 {
              n226 = Wait (ms)(milliseconds to wait=u32 1000) -> ()  [unwired: 1 out]
            }
            frame #1 {
              n227 = Close Reference(reference=w424, error in (no error)=w425) -> ()  [unwired: 1 out]
            }
            frame #2 {
              n228 = Quit LabVIEW() -> ()  [unwired: 1 in]
            }
          }
        }
      }
      n229 = property on="DomainName" class="Str"("Disabled"=u8 0) -> ()  [unwired: 2 in, 2 out]
      n230 = property on="setDomain" class="Bool"("Visible"=TRUE) -> ()  [unwired: 2 in, 2 out]
    }
  }
  n231 = while {
    tunnel: w1 -> [w427]
    stop <- w429 continue-if-true
    n232 = call "DMSU.messages.vi"("Action"=T5."GetMessages") -> ("messages"=w431:string[])  [unwired: 17 in, 1 out]
    n233 = Array Size(array=w431) -> (size(s)=w430:i32)
    n234 = case shown="1, Default" w430 {
      selector: w430 -> [_ w433]
      tunnel: w431 -> [_ w434]
      frame 0 {
      }
      frame 1, Default {
        n235 = property on="Messages" class="LstBox (strict)"() -> ("Item Names"=w438:string[])  [unwired: 2 in, 2 out]
        n236 = Build Array (concatenate)(w434, w438) -> (w436:string[])
        n237 = Array Size(array=w436) -> (size(s)=w437:i32)
        n238 = case shown="0, Default" w437 {
          tunnel: w436 -> [w439 w443]
          tunnel: w433 -> [_ w440]
          tunnel: [w439 w441] -> w435
          frame 0, Default {
          }
          frame 200.. {
            n239 = Delete From Array(array=w443, length=w440, index=200) -> (array with subset deleted=w441:string[])  [unwired: 1 out]
          }
        }
        n240 = property on="Messages" class="LstBox (strict)"("Item Names"=w435) -> ()  [unwired: 2 in, 2 out]
      }
    }
    n241 = Wait on Occurrence(1:FALSE ("ignore previous (T)"), 2:w427, 3:2000 ("ms timeout (-1)")) -> (0:w429:bool)
  }
